vi "String To Number(I16).vi"(5 "String":string) -> (0 "Numeric(I16)":i16)   [LabVIEW 2017]
uses:
  e5ddb552-8b1e-42fe-b921-c4595eeb9d88.vi
  69e60dad-7fd9-4a43-8fe8-3994ebe575b3.vi
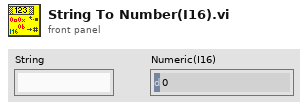
[diagram p1: front panel]
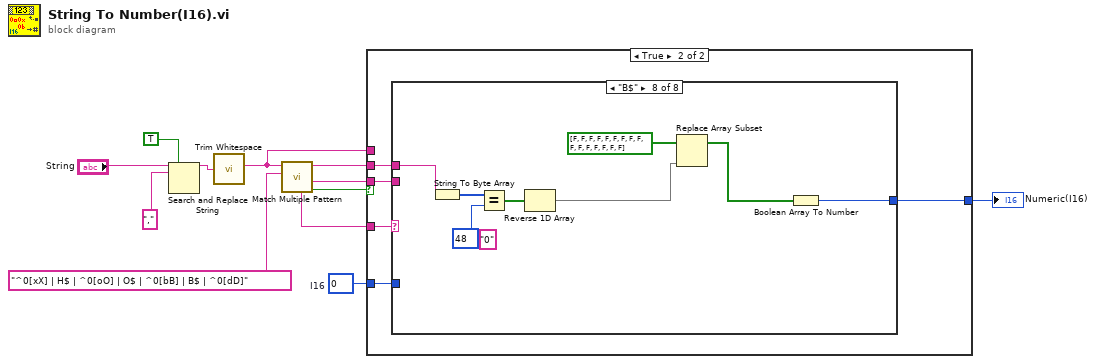
[diagram p0: block diagram]
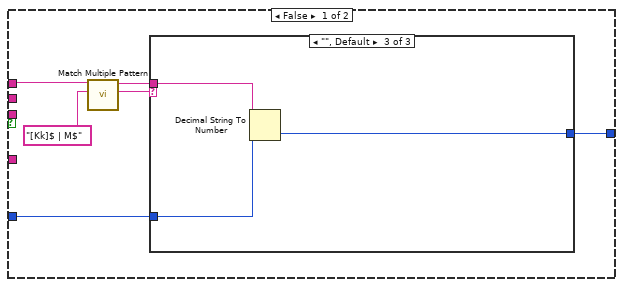
[diagram p2: hidden frame]
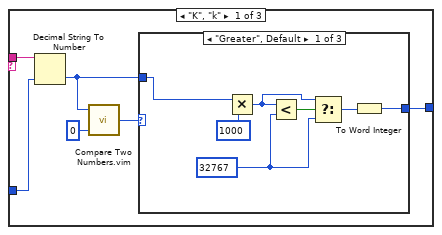
[diagram p3: hidden frame]
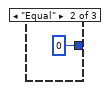
[diagram p4: hidden frame]
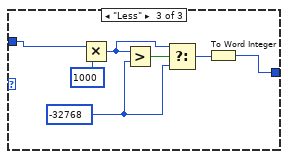
[diagram p5: hidden frame]
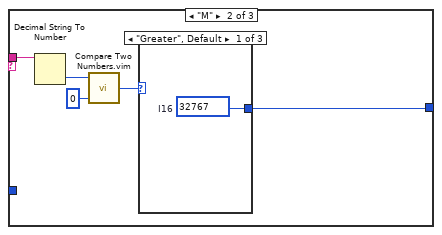
[diagram p6: hidden frame]
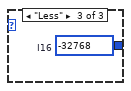
[diagram p8: hidden frame]
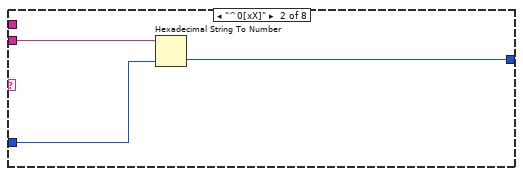
[diagram p10: hidden frame]
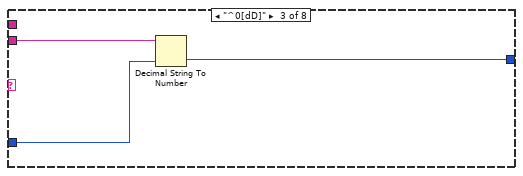
[diagram p11: hidden frame]
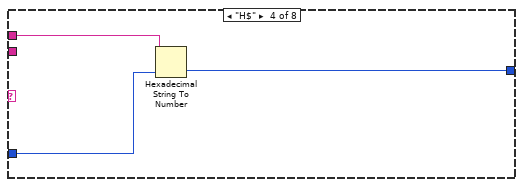
[diagram p12: hidden frame]
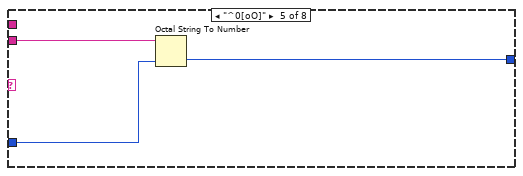
[diagram p13: hidden frame]
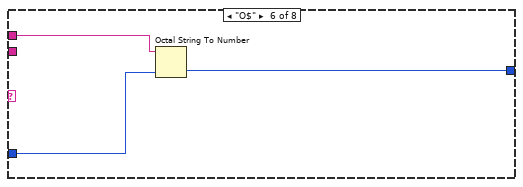
[diagram p14: hidden frame]
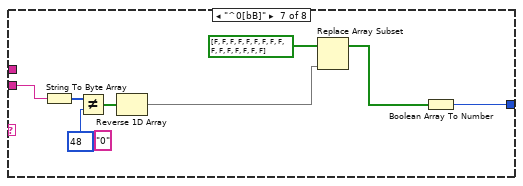
[diagram p15: hidden frame]
diagram:
  w1 = i16 0  # I16
  n1 = Search and Replace String(replace all?=TRUE ("replace all? (F)"), input string="String", search string=",") -> (result string=w9:string)  [unwired: 5 in, 3 out]
  n2 = call <vilib>:"Trim Whitespace.vi"("string"=w9) -> ("trimmed string"=w2:string)  [unwired: 1 in]
  n3 = call "Match Multiple Pattern.vi"("regular expression"="^0[xX] | H$ | ^0[oO] | O$ | ^0[bB] | B$ | ^0[dD]", "string"=w2) -> ("Found?"=w7:bool, "after substring"=w5:string, "before substring"=w4:string, "pattern matched"=w6:string)  [unwired: 5 in, 1 out]
  n4 = case shown="True" w7 {
    tunnel: w6 -> [_ w54]
    tunnel: w5 -> [_ w53]
    tunnel: w4 -> [_ w52]
    tunnel: [w13 w51] -> w3
    tunnel: w2 -> [w14 _]
    tunnel: w1 -> [w15 w50]
    frame False {
      n5 = call "Match Multiple Pattern.vi"("regular expression"="[Kk]$ | M$", "string"=w14) -> ("match substring"=w17:string, "before substring"=w16:string)  [unwired: 5 in, 3 out]
      n6 = case shown="\"\", Default" w17 {
        tunnel: [w21 w40 w49] -> w13
        tunnel: w15 -> [w20 _ w48]
        tunnel: w16 -> [w24 w44 w47]
        frame "K", "k" {
          n7 = Decimal String To Number(string=w24, default (0L)=w20) -> (number=w19:i16)  [unwired: 1 in, 1 out]
          n8 = call "Compare Two Numbers.vim"("Ref"=0, "Number"=w19) -> ("Result"=w22:enum16{"Greater", "Equal", "Less"})  [unwired: 1 in, 2 out]
          n9 = case shown="\"Greater\", Default" w22 {
            tunnel: [w25 i16 0 w33] -> w21
            tunnel: w19 -> [w27 _ w34]
            frame "Greater", Default {
              w28 = i16 32767 ("y")
              n10 = Multiply(x=w27, y=u64 1000) -> (x*y=w29:u64)
              n11 = Less?(x=w29, y=w28) -> (x < y?=w30:bool)
              n12 = Select(t=w29, s=w30, f=w28) -> (s? t:f=w26:u64)
              n13 = To Word Integer(number=w26) -> (16bit integer=w25:i16)
            }
            frame "Equal" {
            }
            frame "Less" {
              w36 = i16 -32768 ("y")
              n14 = Multiply(x=w34, y=u64 1000) -> (x*y=w37:u64)
              n15 = Greater?(x=w37, y=w36) -> (0:w38:bool)
              n16 = Select(t=w37, s=w38, f=w36) -> (s? t:f=w35:u64)
              n17 = To Word Integer(number=w35) -> (16bit integer=w33:i16)
            }
          }
        }
        frame "M" {
          n18 = Decimal String To Number(string=w44) -> (number=w43:i32)  [unwired: 2 in, 1 out]
          n19 = call "Compare Two Numbers.vim"("Ref"=0, "Number"=w43) -> ("Result"=w41:enum16{"Greater", "Equal", "Less"})  [unwired: 1 in, 2 out]
          n20 = case shown="\"Greater\", Default" w41 {
            tunnel: [w45 _ w46] -> w40
            frame "Greater", Default {
              w45 = i16 32767  # I16
            }
            frame "Equal" {
            }
            frame "Less" {
              w46 = i16 -32768  # I16
            }
          }
        }
        frame "", Default {
          n21 = Decimal String To Number(string=w47, default (0L)=w48) -> (number=w49:i16)  [unwired: 1 in, 1 out]
        }
      }
    }
    frame True {
      n22 = case shown="\"B$\"" w54 {
        tunnel: w53 -> [_ w58 w61 _ w67 _ w77 _]
        tunnel: w52 -> [_ _ _ w63 _ w69 _ w83]
        tunnel: [w55 w57 w60 w64 w66 w70 w78 w86] -> w51
        tunnel: w50 -> [w55 w56 w59 w62 w65 w68 _ _]
        frame Default {
        }
        frame "^0[xX]" {
          n23 = Hexadecimal String To Number(string=w58, default (0uL)=w56) -> (number=w57:i16)  [unwired: 1 in, 1 out]
        }
        frame "^0[dD]" {
          n24 = Decimal String To Number(string=w61, default (0L)=w59) -> (number=w60:i16)  [unwired: 1 in, 1 out]
        }
        frame "H$" {
          n25 = Hexadecimal String To Number(string=w63, default (0uL)=w62) -> (number=w64:i16)  [unwired: 1 in, 1 out]
        }
        frame "^0[oO]" {
          n26 = Octal String To Number(2:w65, 4:w67) -> (0:w66:i16)  [unwired: 1 in, 1 out]
        }
        frame "O$" {
          n27 = Octal String To Number(2:w68, 4:w69) -> (0:w70:i16)  [unwired: 1 in, 1 out]
        }
        frame "^0[bB]" {
          (unwired) "0" ("search string")
          n28 = String To Byte Array(string=w77) -> (unsigned byte array=w76:u8[])
          n29 = Not Equal?(x=w76, y=u8 48) -> (x != y?=w74:bool[])
          n30 = Reverse 1D Array(array=w74) -> (reversed array=w72:bool[])
          n31 = Replace Array Subset(array=bool[] [FALSE, FALSE, FALSE, FALSE, FALSE, FALSE, FALSE, FALSE, FALSE, FALSE, FALSE, FALSE, FALSE, FALSE, FALSE, FALSE], new element=w72) -> (w71:bool[])  [unwired: 1 in]
          n32 = Boolean Array To Number(Boolean array=w71) -> (number=w78:i16)
        }
        frame "B$" {
          (unwired) "0" ("search string")
          n33 = String To Byte Array(string=w83) -> (unsigned byte array=w85:u8[])
          n34 = Equal?(x=w85, y=u8 48) -> (x = y?=w84:bool[])
          n35 = Reverse 1D Array(array=w84) -> (reversed array=w80:bool[])
          n36 = Replace Array Subset(array=bool[] [FALSE, FALSE, FALSE, FALSE, FALSE, FALSE, FALSE, FALSE, FALSE, FALSE, FALSE, FALSE, FALSE, FALSE, FALSE, FALSE], new element=w80) -> (w79:bool[])  [unwired: 1 in]
          n37 = Boolean Array To Number(Boolean array=w79) -> (number=w86:i16)
        }
      }
    }
  }
  "Numeric(I16)" <- w3
